vi "Soft_Robot_Model_Conf.vi"() -> ()   [LabVIEW 2015]
uses:
  <vilib>/addons/Control Design/_Stochastic Systems/Stochastic Systems.llb/Stochastic Systems SubVIs/cd_Stochastic State-Space Model.ctl
  <vilib>/addons/Control Design/_Model Construction/Model Typedefs.llb/CD State Space Model (MIMO).ctl
  <vilib>/addons/Control Design/_Model Construction/Model Typedefs.llb/CD General Elements.ctl
  <vilib>/addons/Control Design/_Stochastic Systems/Stochastic Systems.llb/Stochastic Systems SubVIs/cd_Second-Order Statistics Noise Model.ctl
  <vilib>/addons/Control Design/_Stochastic Systems/Stochastic Systems.llb/CD CtoD Stochastic Model.ctl
  <vilib>/Platform/TimedLoop/XDataNode/timing_clust.ctl
  <vilib>/Platform/TimedLoop/XDataNode/nitl_modes.ctl
  <vilib>/Platform/TimedLoop/XDataNode/wakeup.ctl
  <vilib>/addons/Control Design/_Stochastic Systems/Stochastic Systems.llb/CD Construct Stochastic Model (Numeric).vi
  <vilib>/Analysis/7linalg.llb/Create Special Real Matrix.vi
  <vilib>/addons/Control Design/_Stochastic Systems/Stochastic Systems.llb/CD Construct Noise Model (Numeric).vi
  <vilib>/addons/Control Design/_State Feedback Control/State Feedback Control.llb/State Feedback Control SubVis/cd_Linear Quadratic Regulator.vi
  <vilib>/FPGAPlugInAG/myRIO-1900/niLvFpga_Open_myRIO-1900.vi
  <vilib>/rvi/interface/common/dynamic/niFpgaDynamicAddResources.vi
  <vilib>/Utility/error.llb/Error Cluster From Error Code.vi
  <vilib>/rvi/errors/niLvFpgaAdjustHostInterfaceError.vi
  <vilib>/FPGAPlugInAG/Dynamic/niLvFpga_Close_Dynamic.vi
  <vilib>/Simulation/Estimation/Implementation/NILVSim Discrete Kalman Filter.llb/SIM Disc KF Pred and Corr with Pred Gain with Checking Direct LV.vi
  <vilib>/addons/Control Design/_Implementation/CD State Feedback Controller (Multiple Outputs).vi
  <vilib>/Platform/TimedLoop/XDataNode/XDataNode.xnode
  <vilib>/rvi/interface/nirviOpenFPGA/nirviOpenFPGA.xnode
  FPGA Bitfiles/ACC20115_FPGATarget_CurrentControlle_Dt5vFgOzYtY.lvbitx
  Current Controller.vi
  <vilib>/rvi/interface/nirviReadWriteControl/nirviReadWriteControl.xnode
  <vilib>/rvi/interface/nirviCloseFPGA/nirviCloseFPGA.xnode
  <vilib>/Simulation/Implementation/XNodeFramework/SimXNode/SimX.xnode
  <vilib>/addons/Control Design/_State Feedback Control/NI_CD_State Feedback Control.lvlib
  <vilib>/Analysis/NI_AALPro.lvlib
  <vilib>/Platform/TimedLoop/XDataNode/XDNodeRunTimeDep.lvlib
  <vilib>/rvi/interface/Simulation/niFpgaSimulationCallBeginRW.vi
  <vilib>/addons/Control Design/_Stochastic Systems/NI_CD_Stochastic Systems.lvlib
  <vilib>/addons/Control Design/_State-Space Analysis/NI_CD_State-Space Analysis.lvlib
  NiFpgaLv.dll
  <vilib>/addons/Control Design/_Implementation/NI_CD_Implementation.lvlib
  <vilib>/addons/Control Design/_Model Construction/NI_LinSys_Model Typedefs.lvlib
panel:
  in  "SP":dbl(slide)=666.2985074626865 scale=580.0..720.0
  in  "Tab Control":enum32{"Outputs", "SS Outs", "Inputs"}(tab)
  out "Valve Input Current":dbl(graph)
  out "Status?":bool
  out "Detectable?":bool
  out "Observable?":bool
  out "Controllable?":bool
  out "Stabilizable?":bool
  out "Fusion":dbl(graph)
  in  "Current (mA)":i32
  out "KF Posteriori":dbl[](graph)
  out "Plant Output and KF estimation":dbl[][](graph)=[[0.009100087472457918]]
  out "KF Predictor Gain L(k)":dbl[][](array[numeric])=[[1.0]] format="%#.6g"
  out "KF Gain M(k)":dbl[][](array[numeric]) format="%#.6g"
  in  "KF R":dbl[](array[slide])=[0.0009999999999999994] scale=0.001..5000.0
  in  "KF Q":dbl[](array[slide])=[208.24576842493772] scale=0.001..5000.0
  in  "Stop":bool
  in  "LQR R":dbl[](array[slide])=[0.14134702368031526] scale=0.001..5000.0
  in  "LQR Matrix (Q)":dbl[](array[slide])=[1000.0000000000007] scale=0.01..1000.0
  out "LQR Eigenvalues":cdb[](array[numeric]) format="%.5f"
  out "P(k+1|k)":dbl[][](array[numeric])
  out "P(k|k)":dbl[][](array[numeric])
  out "KF Post Value":dbl
  out "Stochastic SS Model":T1={"Sampling Time (s)"=0.0, "G"=[], "B"=[[-1.71e-07], [6.47e-07]], "A"=[], "C"=[], "D"=[], "H"=[]} {"H" format="%#.2g"; "D" format="%#.2g"; "C" format="%#.2g"; "A" format="%#.2g"; "B" format="%#.2g"; "G" format="%#.2g"; "Sampling Time (s)" format="%.2f"}
  out "Deterministic SS Model":T2={"properties"={"Model name"="", "Input names"=[], "Output names"=[], "Input Delays"=[], "Output Delays"=[], "Sampling Time"=0.0, "Notes"=""}, "A"=[], "B"=[[-1.706e-07], [6.469e-07]], "C"=[], "D"=[], "StateNames"=[], "Transport Delay"=[]} {"Transport Delay" format="%.2f"; "D" format="%#.2g"; "C" format="%#.2g"; "B" format="%#.2g"; "A" format="%#.2g"; "properties"."Sampling Time" format="%#.6p"; "properties"."Output Delays" format="%.4f"; "properties"."Input Delays" format="%.4f"}
  out "DAC Loop Error":errorcluster
  out "LQR Error":errorcluster
  out "KF Noise Model":T4 {"N" format="%#.2g"; "R" format="%#.2g"; "E{v}" format="%#.2g"; "E{w}" format="%#.2g"; "Q" format="%#.2g"}
  out "FPGA Loop Error":errorcluster
  out "Control Loop Error":errorcluster
  out "KF Model Error":errorcluster
  out "UDP Loop Error":errorcluster
  in  "A":dbl[][](array[numeric])=[[1.01, -0.1716], [0.001556, 0.9782]] format="%#.5g"
  in  "B":dbl[][](array[numeric])=[[-1.706e-07], [6.469e-07]] format="%#.5g"
  in  "C":dbl[][](array[numeric])=[[1.089, -0.03769]] format="%#.5g"
  in  "G":dbl[][](array[numeric])=[[0.9253], [0.9604]] format="%#.2g"
  in  "xhat(0|-1)":dbl[](array[numeric])=[1.0, 0.0]
  in  "P(0|-1)":dbl[][](array[numeric])=[[1.0, 0.0], [0.0, 1.0]]
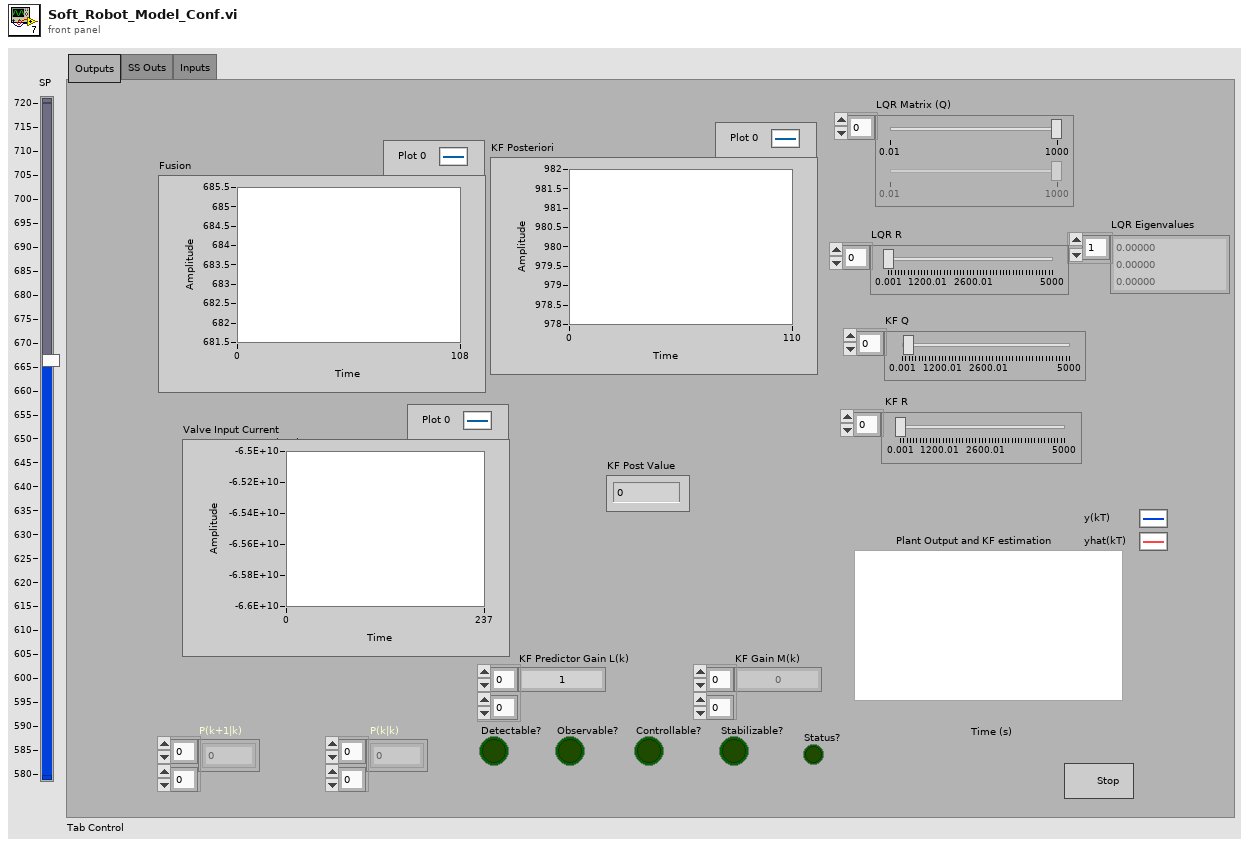
[diagram p1: front panel]
types:
  T1 = typedef "NI_CD_Stochastic Systems.lvlib/cd_Stochastic State-Space Model.ctl" = cluster{"Sampling Time (s)":dbl, "G":dbl[][], "B":dbl[][], "A":dbl[][], "C":dbl[][], "D":dbl[][], "H":dbl[][]}
  T2 = typedef "NI_LinSys_Model Typedefs.lvlib/CD State Space Model (MIMO).ctl" = cluster{"properties":T3, "A":dbl[][], "B":dbl[][], "C":dbl[][], "D":dbl[][], "StateNames":string[], "Transport Delay":dbl[][]}
  T3 = typedef "NI_LinSys_Model Typedefs.lvlib/CD General Elements.ctl" = cluster{"Model name":string, "Input names":string[], "Output names":string[], "Input Delays":dbl[], "Output Delays":dbl[], "Sampling Time":dbl, "Notes":string}
  T4 = typedef "NI_CD_Stochastic Systems.lvlib/cd_Second-Order Statistics Noise Model.ctl" = cluster{"Q":dbl[][], "E{w}":dbl[], "E{v}":dbl[], "R":dbl[][], "N":dbl[][]}
  T5 = enum32{"Identity", "Diagonal", "Toepliz", "Vandermonde", "Companion"}
  T6 = typedef "NI_CD_Stochastic Systems.lvlib/CD CtoD Stochastic Model.ctl" = enum16{"Truncation of Taylor Series", "Numerical Integration"}
  T7 = enum16{"state weighting", "output weighting, Dim Q = Ny", "output weighting, Dim Q = Nx"}
  T8 = typedef "NI_Matrix.lvlib/RealMatrix.ctl" = dbl[][]
  T9 = typedef "XDNodeRunTimeDep.lvlib/timing_clust.ctl" = cluster{"Expected End [f-1]":u64, "Actual End [f-1]":u64, "Finished Late? [f-1]":bool, "Expected End [i-1]":u64, "Actual End [i-1]":u64, "Finished Late? [i-1]":bool, "Expected Start [i]":u64, "Actual Start [i]":u64, "Expected Start [f]":u64, "Actual Start [f]":u64, "Source Name":string, "Structure Name":string, "Period":i64, "Deadline":i64, "Offset":i64, "Start":i64, "Priority":i32, "Timeout":i32, "Mode":T10, "Wakeup Reason":T11, "Error":errorcluster, "Source Type":string, "Secondary Source Type":string, "Global End Time":u64, "Global Start Time":u64, "Frame Duration":u64, "Iteration Duration":u64, "Assigned CPU":i32, "I/O Scan Engine Mode":u32}
  T10 = typedef "XDNodeRunTimeDep.lvlib/nitl_modes.ctl" = enum32{"No Change", "Process missed periods, maintain original phase", "Discard missed periods, maintain original phase", "Process missed periods, ignore original phase", "Discard missed periods, ignore original phase"}
  T11 = typedef "XDNodeRunTimeDep.lvlib/wakeup.ctl" = enum32{"Normal", "Aborted", "Asynchronous wakeup", "Timing source error", "Timed loop error", "Timeout"}
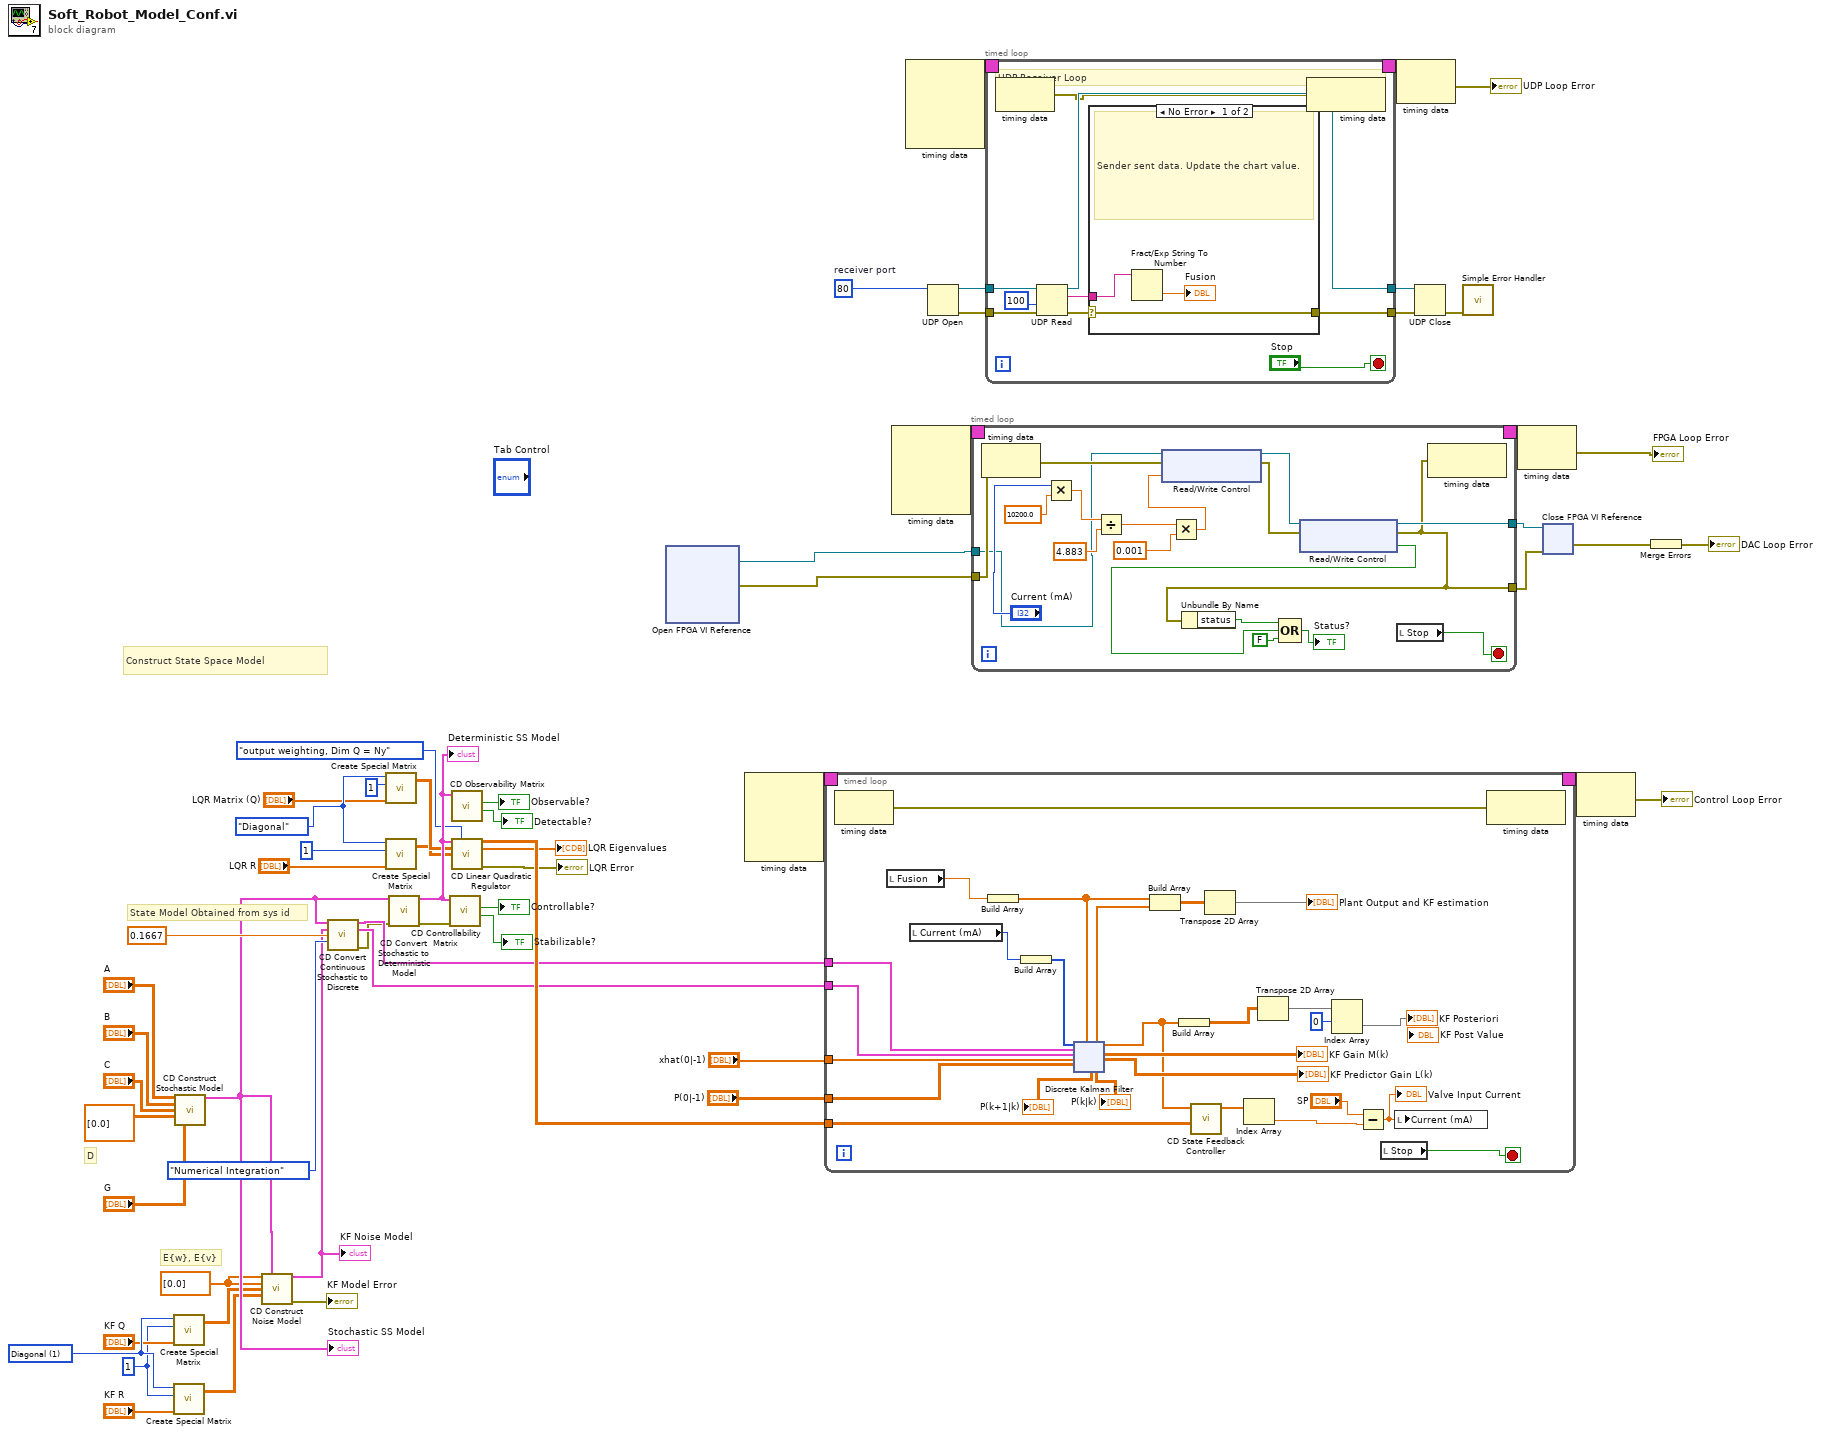
[diagram p0: block diagram]
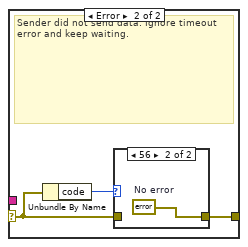
[diagram p2: hidden frame]
diagram:
  w6 = T5."Diagonal" ("matrix type")
  w7 = 1 ("KF Q/R Size")
  w11 = dbl[] [0.0] ("E{w}")
  w12 = 1 items=["Identity", "Diagonal", "Toeplitz", "Vandermonde", "Companion", "Hankel", "Hadamard", "Wilkinson", "Hilbert", "Inverse Hilbert", "Rosser", "Pascal"] ("matrix type")
  w48 = u16 80  # receiver port
  # "E{w}, E{v}"
  # "D"
  # "State Model Obtained from sys id"
  # "Construct State Space Model"
  n1 = call-poly <vilib>:"Create Special Matrix.vi"("matrix type"=w12, "matrix size"=w7, "Input Vector1"="KF Q") -> ("Special Matrix"=w14:T8)  [unwired: 2 in, 1 out]
  n2 = call-poly <vilib>:"Create Special Matrix.vi"("matrix type"=w12, "matrix size"=w7, "Input Vector1"="KF R") -> ("Special Matrix"=w13:T8)  [unwired: 2 in, 1 out]
  n3 = call-poly <vilib>:"CD Construct Stochastic Model.vi"("A"="A", "B"="B", "C"="C", "D"=dbl[][] [[0.0]], "G"="G") -> ("Stochastic State-Space Model"=w27:T1)  [unwired: 3 in, 7 out]
  "Stochastic SS Model" <- w27
  n4 = call-poly <vilib>:"CD Construct Noise Model.vi"("E{w}"=w11, "Stochastic State-Space Model"=w27, "E{v}"=w11, "Q"=w14, "R"=w13) -> ("Second-Order Statistics Noise Model out"=w28:T4, "error out"=→"KF Model Error":errorcluster)  [unwired: 2 in, 7 out]
  "KF Noise Model" <- w28
  n5 = call <vilib>:"CD Convert Continuous Stochastic to Discrete.vi"("Continuous Stochastic\nState-Space Model"=w27, "Continuous Second-Order\nStatistics Noise Model"=w28, "Sampling Time (s)"=0.1667, "Method"=CD_CtoD_Stochastic_Model."Numerical Integration") -> ("Discrete Stochastic\nState-Space Model"=w37:T1, "Discrete Second-Order\nStatistics Noise Model"=w38:T4, "error out"=w22:errorcluster)  [unwired: 1 in, 8 out]
  n6 = call-poly <vilib>:"Create Special Matrix.vi"("matrix type"=w6, "matrix size"=1, "Input Vector1"="LQR Matrix (Q)") -> ("Special Matrix"=w18:T8)  [unwired: 2 in, 1 out]
  n7 = call-poly <vilib>:"Create Special Matrix.vi"("matrix type"=w6, "matrix size"=1, "Input Vector1"="LQR R") -> ("Special Matrix"=w15:T8)  [unwired: 2 in, 1 out]
  n8 = call <vilib>:"CD Convert Stochastic to Deterministic Model.vi"("Stochastic State-Space Model"=w27, "error in (no error)"=w22) -> ("Deterministic State-Space Model"=w36:T2, "error out"=w21:errorcluster)  [unwired: 12 in]
  "Deterministic SS Model" <- w36
  n9 = call <vilib>:"CD Controllability Matrix.vi"("error in (no error)"=w21, "State-Space Model"=w36) -> ("Is Stabilizable?"=→"Stabilizable?":bool, "Is Controllable?"=→"Controllable?":bool)  [unwired: 6 in, 2 out]
  n10 = call <vilib>:"CD Observability Matrix.vi"("State-Space Model"=w36) -> ("Is Detectable?"=→"Detectable?":bool, "Is Observable?"=→"Observable?":bool)  [unwired: 7 in, 2 out]
  n11 = call-poly <vilib>:"CD Linear Quadratic Regulator.vi"("State-Space Model"=w36, "Weighting Type"=T7."output weighting, Dim Q = Ny", "Q"=w18, "R"=w15) -> ("Optimal Gain (K)"=w39:dbl[][], "Eigenvalues"=→"LQR Eigenvalues":cdb[], "error out"=→"LQR Error":errorcluster)  [unwired: 8 in, 1 out]
  n12 = xnode "Open FPGA VI Reference"() -> ("FPGA VI Reference Out"=w47:refnum<k20>, "error out"=w46:errorcluster)  [unwired: 2 in]
  n13 = node-c288() -> (w41:T9)  [unwired: 4 in]
  n14 = timed-loop {
    timing: w41 -> [_]
    timing-out: [_] -> w40
    tunnel: w39 -> [w63]
    tunnel: w38 -> [w87]
    tunnel: w37 -> [w66]
    tunnel: "xhat(0|-1)" -> [w86]
    tunnel: "P(0|-1)" -> [w85]
    stop <- w61 stop-if-true
    n15 = node-c288() -> (w71:errorcluster)  [unwired: 1 in]
    n16 = local read "Fusion"() -> (w73:dbl)
    n17 = local read "Current (mA)"() -> (w72:i32)
    n18 = Build Array ("Build Array 3")(w73) -> (w76:dbl[])
    n19 = Build Array ("Build Array 5")(w72) -> (w83:i32[])
    n20 = xnode ("Discrete Kalman Filter")("input u(k)"=w83, "Stochastic State-Space Model"=w66, "Second-Order Statistics Noise Model"=w87, "Initial State Estimate xhat(0|-1)"=w86, "Initial Estimation Error Covariance P(0|-1)"=w85, "Output y(k)"=w76) -> ("Prediction Error Covariance P(k+1|k)"=→"P(k+1|k)":dbl[][], "Estimated Output yhat(k)"=w82:dbl[], "Filter Error Covariance P(k|k)"=→"P(k|k)":dbl[][], "Corrected State Estimate xhat(k|k)"=w77:dbl[], "Kalman Filter Gain M(k)"=→"KF Gain M(k)":dbl[][], "Kalman Predictor Gain L(k)"=→"KF Predictor Gain L(k)":dbl[][])  [unwired: 2 in, 2 out]
    n21 = Build Array(w76, w82) -> (w81:dbl[][])
    n22 = Build Array ("Build Array 2")(w77) -> (w69:dbl[][])
    n23 = call-poly <vilib>:"CD State Feedback Controller.vi"("Controller Gain"=w63, "States"=w77) -> ("Controller Action"=w84:dbl[])  [unwired: 8 in, 1 out]
    n24 = Transpose 2D Array(2D array=w81) -> (transposed array=→"Plant Output and KF estimation":dbl[][])
    n25 = Index Array(array=w84) -> (element=w74:dbl)  [unwired: 1 in]
    n26 = Transpose 2D Array(2D array=w69) -> (transposed array=w68:dbl[][])
    n27 = Index Array(array=w68, index (row)=0) -> (element=→"KF Posteriori":dbl[])  [unwired: 1 in]
    n28 = Subtract ("Subtract 2")(x="SP", y=w74) -> (x-y=w67:dbl)
    "Valve Input Current" <- w67
    n29 = local read "Stop"() -> (w61:bool)
    n30 = local write "Current (mA)"(w67) -> ()
    n31 = node-c288(w71) -> ()  [unwired: 1 out]
  }
  n32 = node-c288() -> (w58:T9)  [unwired: 4 in]
  n33 = node-c288() -> (w45:T9)  [unwired: 4 in]
  n34 = UDP Open(11:w48) -> (port=w49:refnum<k16>, 0:w50:errorcluster)  [unwired: 4 in, 1 out]
  n35 = timed-loop {
    tunnel: w46 -> [w112]
    tunnel: [w111] -> w56
    tunnel: [w120] -> w60
    timing: w58 -> [_]
    timing-out: [_] -> w57
    tunnel: w47 -> [w110]
    stop <- w109 stop-if-true
    n36 = node-c288() -> ()  [unwired: 1 in, 1 out]
    n37 = Multiply(x="Current (mA)", y=10200.0) -> (x*y=w115:dbl)
    n38 = Divide(x=w115, y=4.883) -> (x/y=w118:dbl)
    n39 = Multiply(x=w118, y=0.001) -> (x*y=w114:dbl)
    n40 = xnode "Read/Write Control"("FPGA VI Reference In"=w110, "error in"=w112, "DAC Inlet Valve"=w114) -> ("FPGA VI Reference Out"=w126:refnum<k20>, "error out"=w125:errorcluster)
    n41 = xnode "Read/Write Control"("FPGA VI Reference In"=w126, "error in"=w125) -> ("FPGA VI Reference Out"=w120:refnum<k20>, "error out"=w111:errorcluster, "Inlet Overflow?"=w121:bool)
    n42 = Unbundle By Name(w111) -> ("status"=w123:bool)
    n43 = Compound Arithmetic op=OR(w123, w121, FALSE ("value")) -> (→"Status?":bool)
    n44 = local read "Stop"() -> (w109:bool)
    n45 = node-c288(w111) -> ()  [unwired: 1 out]
  }
  n46 = timed-loop {
    tunnel: w49 -> [w139]
    tunnel: [w133] -> w53
    tunnel: w50 -> [w138]
    tunnel: [w134] -> w51
    timing: w45 -> [_]
    timing-out: [_] -> w44
    stop <- "Stop" stop-if-true
    # "UDP Receiver Loop"
    n47 = node-c288() -> (w131:errorcluster)  [unwired: 1 in]
    n48 = UDP Read(connection ID=w139, timeout ms (25000)=100, 8:w138) -> (data out=w136:string, error out=w135:errorcluster, 3:w133:refnum<k16>)  [unwired: 3 out]
    n49 = case shown="No Error" w135 {
      selector: w135 -> [w145 w149]
      tunnel: w136 -> [w147 _]
      tunnel: [w145 w148] -> w134
      frame No Error {
        # "Sender sent data. Update the chart value."
        n50 = Fract/Exp String To Number(string=w147) -> (number=→"Fusion":dbl)  [unwired: 3 in, 1 out]
      }
      frame Error {
        # "Sender did not send data. Ignore timeout error and keep waiting."
        n51 = Unbundle By Name(w149) -> ("code"=w150:i32)
        n52 = case shown="56" w150 {
          tunnel: w149 -> [w151 _]
          tunnel: [w151 w152] -> w148
          frame Default {
          }
          frame 56 {
            w152 = errorcluster {"status"=FALSE, "code"=0, "source"=""}  # No error
          }
        }
      }
    }
    n53 = node-c288(w131) -> ()  [unwired: 1 out]
  }
  n54 = node-c288(w44) -> (→"UDP Loop Error":errorcluster)
  n55 = UDP Close(connection ID=w53, 8:w51) -> (error out=w52:errorcluster)  [unwired: 1 out]
  n56 = call <vilib>:"Simple Error Handler.vi"("error in (no error)"=w52) -> ()  [unwired: 1 in, 8 out]
  n57 = node-c288(w57) -> (→"FPGA Loop Error":errorcluster)
  n58 = xnode "Close FPGA VI Reference"("FPGA VI Reference In"=w60, "error in"=w56) -> ("error out"=w55:errorcluster)
  n59 = node-c288(w40) -> (→"Control Loop Error":errorcluster)
  n60 = Merge Errors(w55) -> (→"DAC Loop Error":errorcluster)
